vi "Insert SSM and SDI.vi"(9 "SSM":u32, 10 "SDI":u32, 11 "Hex (in)":string="AAAAAAAA") -> (3 "Hex (out)":string)   [LabVIEW 2017]
panel:
  out "Decimal (out)":u32
  out "Boolean Array (out)":bool[](array[boolean])
  out "SSM":bool[](array[boolean])
  out "SDI":bool[](array[boolean])
  out "Boolean Array (in)":bool[](array[boolean])
  out "Decimal (in)":u32
  # "Bit 32"
  # "Bit 0"
  # "Bit 32"
  # "Bit 0"
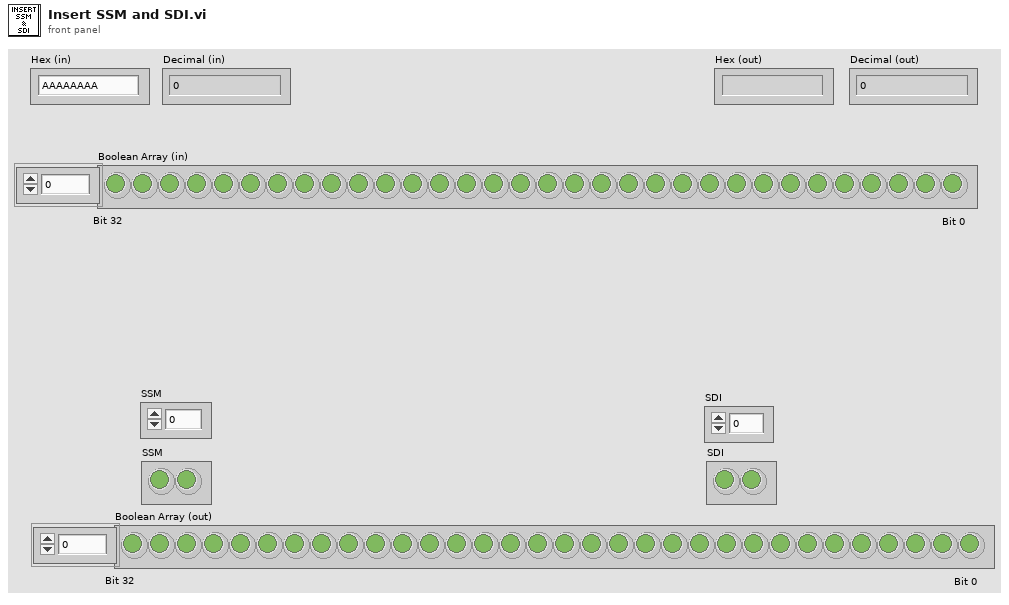
[diagram p1: front panel]
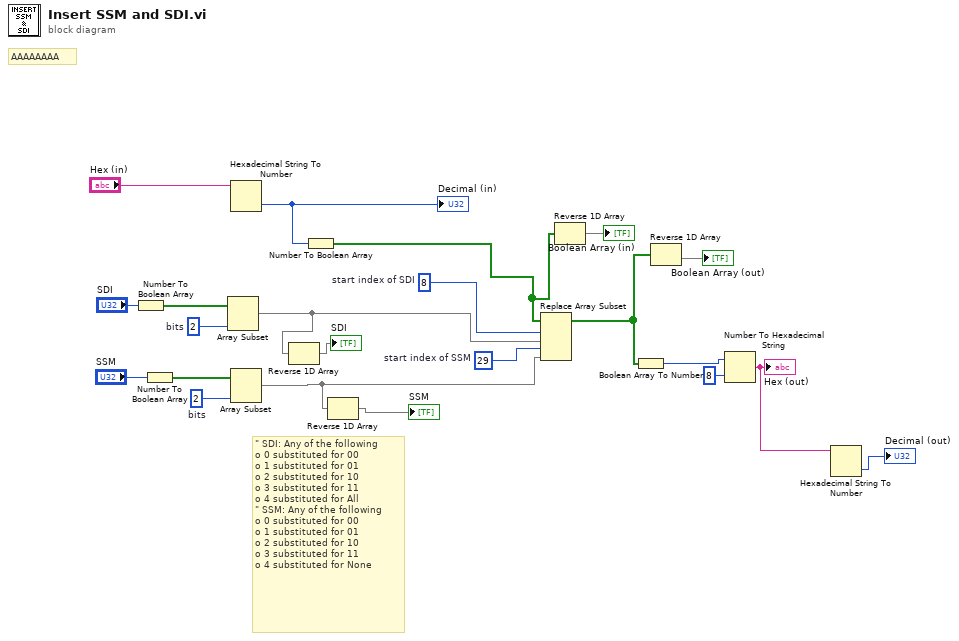
[diagram p0: block diagram]
diagram:
  w14 = 29  # start index of SSM
  w15 = 8  # start index of SDI
  w17 = 2  # bits
  w18 = 2  # bits
  # "\"\tSDI: Any of the following \no\t0 substituted for 00\no\t1 substituted for 01\no\t2 substituted for 10\no\t3 substituted for 11\no\t4 substituted for All\n\"\tSSM: Any of the following \no\t0 substituted for 00\no\t1 substituted for 01\no\t2 substituted for 10\no\t3 substituted for 11\no\t4 substituted for None"
  # "AAAAAAAA"
  n1 = Number To Boolean Array(number="SDI") -> (Boolean array=w13:bool[])
  n2 = Number To Boolean Array(number="SSM") -> (Boolean array=w16:bool[])
  n3 = Array Subset(array=w13, length=w18) -> (w8:bool[])  [unwired: 1 in]
  n4 = Hexadecimal String To Number(string="Hex (in)") -> (number=w21:u32)  [unwired: 2 in, 1 out]
  "Decimal (in)" <- w21
  n5 = Array Subset(array=w16, length=w17) -> (w6:bool[])  [unwired: 1 in]
  n6 = Reverse 1D Array(array=w8) -> (reversed array=→"SDI":bool[])
  n7 = Number To Boolean Array(number=w21) -> (Boolean array=w4:bool[])
  n8 = Reverse 1D Array(array=w6) -> (reversed array=→"SSM":bool[])
  n9 = Replace Array Subset(array=w4, new element #1=w8, index #1=w15, new element #2=w6, index #2=w14) -> (w2:bool[])
  n10 = Reverse 1D Array(array=w4) -> (reversed array=→"Boolean Array (in)":bool[])
  n11 = Boolean Array To Number(Boolean array=w2) -> (number=w12:u32)
  n12 = Reverse 1D Array(array=w2) -> (reversed array=→"Boolean Array (out)":bool[])
  n13 = Number To Hexadecimal String(1:i16 8 ("width (-)"), 2:w12) -> (0:w10:string)
  "Hex (out)" <- w10
  n14 = Hexadecimal String To Number(string=w10) -> (number=→"Decimal (out)":u32)  [unwired: 2 in, 1 out]
